vi "ELVIS III v1.0 Reserve AO Continuous.vi"(8 "error in (no error)":errorcluster, 11 "AO (Continuous) Channels List":T2 caption="AI (N Samples) Channels List") -> (0 "error out":errorcluster, 3 "Channel Info":T1)   [LabVIEW 2021]
uses:
  <vilib>/myRIO/Common/Instrument Driver Framework/ELVIS III v1.0/AO Continuous/typedefs/AO Continuous Channels List.ctl
  <vilib>/myRIO/Common/Instrument Driver Framework/ELVIS III v1.0/AO Continuous/typedefs/ELVIS III v1.0 AO Continuous Channels Enum.ctl
  <vilib>/myRIO/Common/Instrument Driver Framework/ELVIS III v1.0/AO Continuous/typedefs/AO Continuous Channel Info.ctl
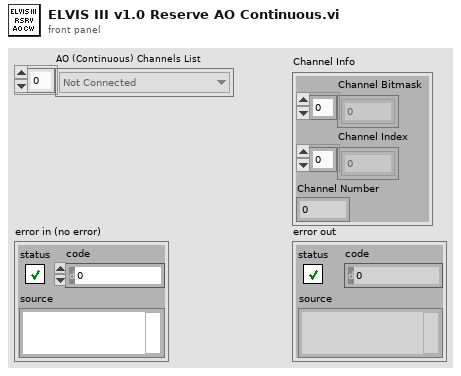
[diagram p1: front panel]
types:
  T1 = typedef "AO Continuous Channel Info.ctl" = cluster{"Channel Bitmask":u8[], "Channel Index":i32[], "Channel Number":u8}
  T2 = typedef "AO Continuous Channels List.ctl" = T3[]
  T3 = typedef "ELVIS III v1.0 AO Continuous Channels Enum.ctl" = enum16{"Not Connected", "A/AO0 (Continuous)", "A/AO1 (Continuous)", "B/AO0 (Continuous)", "B/AO1 (Continuous)"}
  T4 = typedef "ELVIS III v1.0 Channel Reservation List.ctl" = T5[]
  T5 = typedef "ELVIS III v1.0 Channel Reservation Info.ctl" = cluster{"Channel Name":string, "Connector":T6, "MutexIDs":u32[]}
  T6 = typedef "ELVIS III v1.0 Connector List.ctl" = enum32{"None", "ConnectorA", "ConnectorB"}
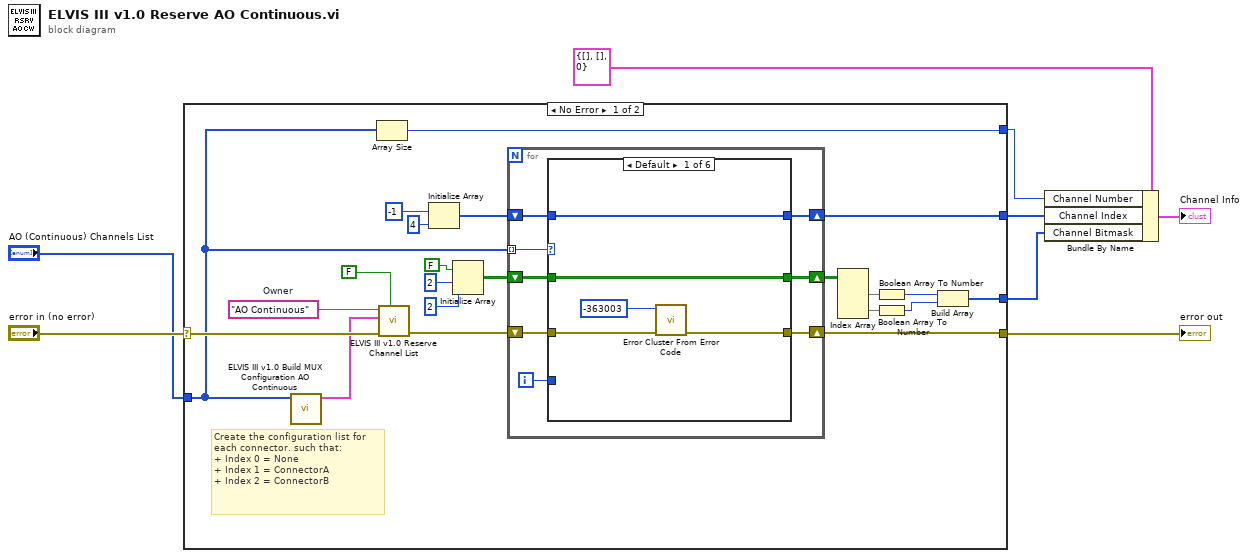
[diagram p0: block diagram]
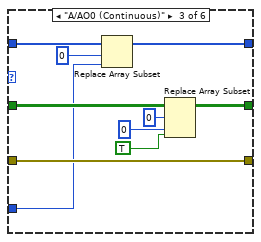
[diagram p3: hidden frame]
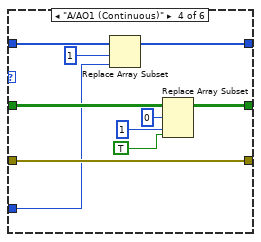
[diagram p4: hidden frame]
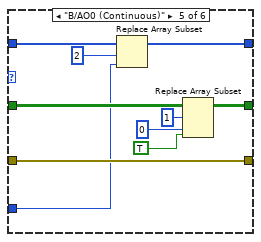
[diagram p5: hidden frame]
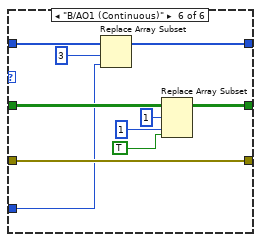
[diagram p6: hidden frame]
diagram:
  n1 = case shown="No Error" "error in (no error)" {
    selector: "error in (no error)" -> [w30 w87]
    tunnel: [w25 w87] -> w8
    tunnel: "AO (Continuous) Channels List" -> [w10 _]
    tunnel: [w15 _] -> w5
    tunnel: [w11 _] -> w4
    tunnel: [w9 _] -> w1
    frame No Error {
      w28 = "AO Continuous"  # Owner
      # "Create the configuration list for each connector. such that:\n+ Index 0 = None\n+ Index 1 = ConnectorA\n+ Index 2 = ConnectorB"
      n2 = call <vilib>:"ELVIS III v1.0 Build MUX Configuration AO Continuous.vi"("AO (Continuous) Channels List"=w10) -> ("Channel Reservation Info"=w29:T4)  [unwired: 10 in]
      n3 = Array Size(array=w10) -> (size(s)=w9:i32)
      n4 = call <vilib>:"ELVIS III v1.0 Reserve Channel List.vi"("Allow multiple opens?"=FALSE, "error in (no error)"=w30, "Channel Reservation List"=w29, "Owner"=w28) -> ("error out"=w26:errorcluster)  [unwired: 7 in]
      n5 = Initialize Array(i8 -1, 4 ("dimension size")) -> (w12:i8[])
      n6 = Initialize Array(FALSE ("element"), 2 ("dimension size"), 2 ("dimension size")) -> (w21:bool[][])
      n7 = for {
        tunnel: w10 -> [w38] mode=indexing
        shift-right: [w36] -> w20
        shift-left: w21 -> [w37]
        shift-right: [w34] -> w25
        shift-left: w26 -> [w35]
        shift-right: [w31] -> w11
        shift-left: w12 -> [w33]
        i -> [w32]
        n8 = case shown="Default" w38 {
          tunnel: w37 -> [w40 w46 w52 w62 w73 w83]
          tunnel: [w40 w46 w53 w63 w72 w82] -> w36
          tunnel: w35 -> [w42 w45 w51 w61 w71 w81]
          tunnel: [w41 w45 w51 w61 w71 w81] -> w34
          tunnel: w33 -> [w39 w44 w50 w59 w69 w79]
          tunnel: w32 -> [_ _ w48 w58 w68 w78]
          tunnel: [w39 w44 w47 w57 w67 w77] -> w31
          frame Default {
            n9 = call <vilib>:"Error Cluster From Error Code.vi"("error in (no error)"=w42, "error code (0)"=-363003) -> ("error out"=w41:errorcluster)  [unwired: 7 in]
          }
          frame "Not Connected" {
          }
          frame "A/AO0 (Continuous)" {
            n10 = Replace Array Subset(array=w50, new element=w48, index=0) -> (w47:i8[])
            n11 = Replace Array Subset(array=w52, new element=TRUE ("new element/subarray"), index (row)=0 ("index"), index (col)=0 ("disabled index (col)")) -> (w53:bool[][])
          }
          frame "A/AO1 (Continuous)" {
            n12 = Replace Array Subset(array=w59, new element=w58, index=1) -> (w57:i8[])
            n13 = Replace Array Subset(array=w62, new element=TRUE ("new element/subarray"), index (row)=0 ("index"), index (col)=1 ("disabled index (col)")) -> (w63:bool[][])
          }
          frame "B/AO0 (Continuous)" {
            n14 = Replace Array Subset(array=w69, new element=w68, index=2) -> (w67:i8[])
            n15 = Replace Array Subset(array=w73, new element=TRUE ("new element/subarray"), index (row)=1 ("index"), index (col)=0 ("disabled index (col)")) -> (w72:bool[][])
          }
          frame "B/AO1 (Continuous)" {
            n16 = Replace Array Subset(array=w79, new element=w78, index=3) -> (w77:i8[])
            n17 = Replace Array Subset(array=w83, new element=TRUE ("new element/subarray"), index (row)=1 ("index"), index (col)=1 ("disabled index (col)")) -> (w82:bool[][])
          }
        }
      }
      n18 = Index Array(array=w20) -> (element #1=w19:bool[], element #2=w18:bool[])  [unwired: 4 in]
      n19 = Boolean Array To Number(Boolean array=w19) -> (number=w17:u8)
      n20 = Boolean Array To Number(Boolean array=w18) -> (number=w16:u8)
      n21 = Build Array(w17, w16) -> (w15:u8[])
    }
    frame Error {
      # "There is an incoming error so there is nothing to do."
    }
  }
  "error out" <- w8
  n22 = Bundle By Name(cluster=T1 {"Channel Bitmask"=[], "Channel Index"=[], "Channel Number"=0} ("Channel Info"), "Channel Number"=w1, "Channel Index"=w4, "Channel Bitmask"=w5) -> (→"Channel Info":T1)
